vi "ExtendedKalmanFilter_New.vi"(5 "States":i32, 6 "UNSCENTED_KALMAN_FUNC_GROUP":T1, 7 "Inputs":i32, 8 "dt_Seconds":dbl=0.02, 9 "MeasurementStdDevs":T3, 10 "StateStdDevs":T3, 11 "Outputs":i32) -> (0 "Error":bool, 3 "UnscentedKalmanFiilter":T4)   [LabVIEW 2019, in "Trajectory_Library.lvlib"]
doc: "Creates a new LINEAR SYSTEM data cluster with the specified values. \n\n\nInputs: \n - XXX -- XXX.\n\nOutputs:\n - XXX -- XXX."
uses:
  Trajectory_Library.lvlib
  EXTENDED_KALMAN_FILTER.ctl
  <vilib>/Analysis/Matrix/Datatypes/RealMatrix.ctl
  EXTENDED_KALMAN_CORRECT_FUNC_GROUP.ctl
  BiFun_Matrix_FUNC_TYPE.ctl
  <vilib>/Analysis/7linalg.llb/Real Transpose Matrix.vi
  <vilib>/Analysis/baseanly.llb/A x B.vi
  <vilib>/Analysis/baseanly.llb/Real A x B.vi
  Discretization_DiscretizeA.vi
  <vilib>/Analysis/Matrix/Numeric/Add/Add.vi
  <vilib>/Analysis/Matrix/Numeric/Add/Add - RM,RM.vi
  <vilib>/Analysis/Matrix/Numeric/Multiply/Multiply.vi
  <vilib>/Analysis/Matrix/Numeric/Multiply/Multiply - RM,R.vi
  Matrix_Exp.vi
  <vilib>/Analysis/Matrix/NI_Matrix.lvlib
  <vilib>/Analysis/NI_AALPro.lvlib
panel:
  # "<States,1>"
  # "<Outputs,1>"
  # "State Estimate <Statess,1>"
  # "<States, States>"
  # "<States, States>"
  # "<Statess,  States>"
  # "<Outputs, Outputs>"
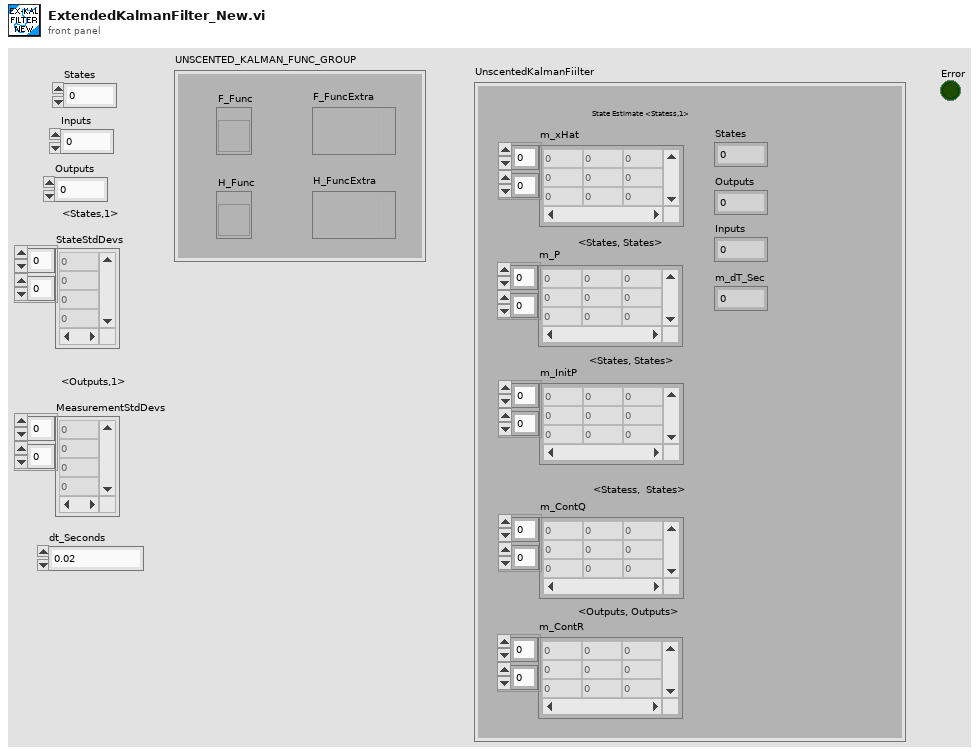
[diagram p1: front panel]
types:
  T1 = typedef "EXTENDED_KALMAN_CORRECT_FUNC_GROUP.ctl" = cluster{"H_Func":T2, "F_Func":T2, "H_FuncExtra":variant, "F_FuncExtra":variant}
  T2 = typedef "Trajectory_Library.lvlib/BiFun_Matrix_FUNC_TYPE.ctl" = refnum<vi>
  T3 = typedef "NI_Matrix.lvlib/RealMatrix.ctl" = dbl[][]
  T4 = typedef "Trajectory_Library.lvlib/EXTENDED_KALMAN_FILTER.ctl" = cluster{"m_P":T3, "m_xHat":T3, "States":i32, "Outputs":i32, "m_ContR":T3, "m_ContQ":T3, "m_dT_Sec":dbl, "Inputs":i32, "m_InitP":T3}
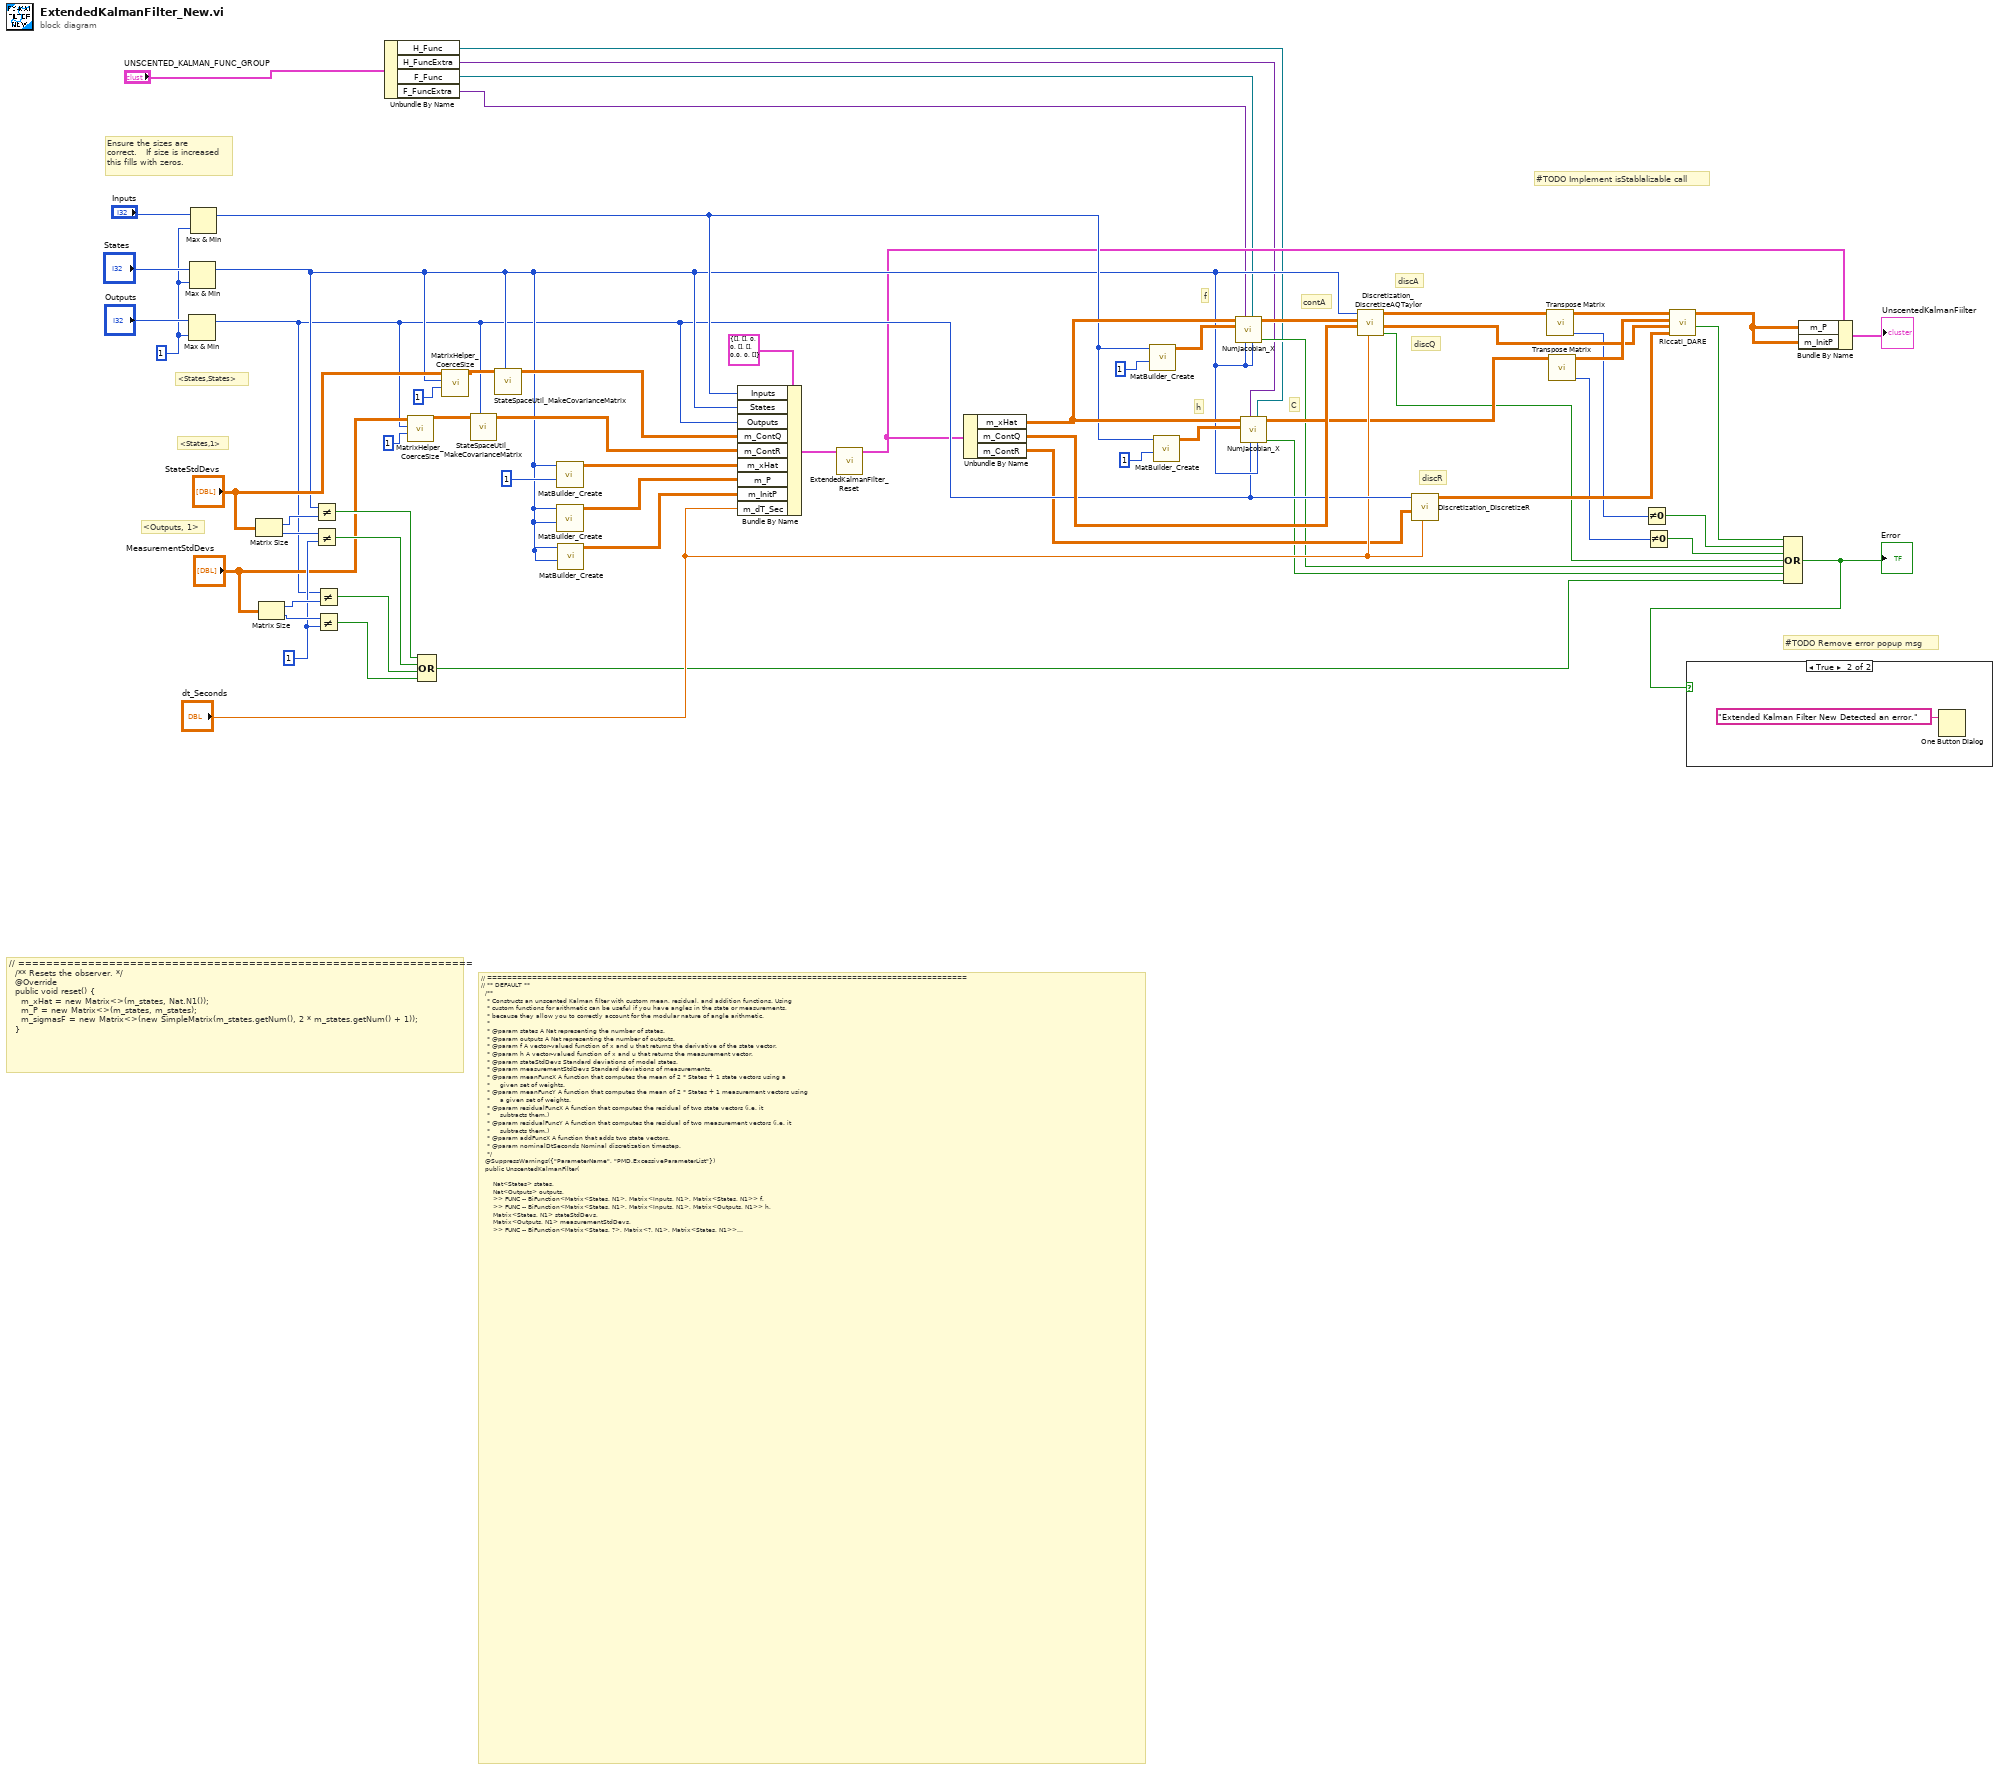
[diagram p0: block diagram]
diagram:
  w53 = 1 ("y")
  w47 = 1 ("y")
  # "#TODO Implement isStablalizable call"
  # "discR"
  # "discQ"
  # "discA"
  # "C"
  # "contA"
  # "h"
  # "f"
  # "// =================================================================\n  /** Resets the observer. */\n  @Override\n  public void reset() {\n    m_xHat = new Matrix<>(m_states, Nat.N1());\n    m_P = new Matrix<>(m_states, m_states);\n    m_sigmasF = new Matrix<>(new SimpleMatrix(m_states.getNum(), 2 * m_states.getNum() + 1));\n  }"
  # "// ================================================================================================\n// ** DEFAULT **\n  /**\n   * Constructs an unscented Kalman filter with custom mean, residual, and addition functions. Using\n   * custom functions for arithmetic can be useful if you have angles in the state or measurements,\n   * because they allow you to correctly account for the modular nature of angle arithmetic.\n   *\n   * @param states A Nat representing the number of states.\n   * @param outputs A Nat representing the number of outputs.\n   * @param f A vector-valued function of x and u that returns the derivative of the state vector.\n   * @param h A vector-valued function of x and u that returns the measurement vector.\n   * @param stateStdDevs Standard deviations of model states.\n   * @param measurementStdDevs Standard deviations of measurements.\n   * @param meanFuncX A function that computes the mean of 2 * States + 1 state vectors using a\n   *     given set of weights.\n   * @param meanFuncY A function that computes the mean of 2 * States + 1 measurement vectors using\n   *     a given set of weights.\n   * @param residualFuncX A function that computes the residual of two state vectors (i.e. it\n   *     subtracts them.)\n   * @param residualFuncY A function that computes the residual of two measurement vectors (i.e. it\n   *     subtracts them.)\n   * @param addFuncX A function that adds two state vectors.\n   * @param nominalDtSeconds Nominal discretization timestep.\n   */\n  @SuppressWarnings({\"ParameterName\", \"PMD.ExcessiveParameterList\"})\n  public UnscentedKalmanFilter(\n\n      Nat<States> states,\n      Nat<Outputs> outputs,\n      >> FUNC -- BiFunction<Matrix<States, N1>, Matrix<Inputs, N1>, Matrix<States, N1>> f,\n      >> FUNC -- BiFunction<Matrix<States, N1>, Matrix<Inputs, N1>, Matrix<Outputs, N1>> h,\n      Matrix<States, N1> stateStdDevs,\n      Matrix<Outputs, N1> measurementStdDevs,\n      >> FUNC -- BiFunction<Matrix<States, ?>, Matrix<?, N1>, Matrix<States, N1>> meanFuncX,\n      >> FUNC -- BiFunction<Matrix<Outputs, ?>, Matrix<?, N1>, Matrix<Outputs, N1>> meanFuncY,\n      >> FUNC -- BiFunction<Matrix<States, N1>, Matrix<States, N1>, Matrix<States, N1>> residualFuncX,\n      >> FUNC -- BiFunction<Matrix<Outputs, N1>, Matrix<Outputs, N1>, Matrix<Outputs, N1>> residualFuncY,\n      >> FUNC -- BiFunction<Matrix<States, N1>, Matrix<States, N1>, Matrix<States, N1>> addFuncX,\n      double nominalDtSeconds) {\n\n    this.m_states = states;\n    this.m_outputs = outputs;\n\n    m_f = f;\n    m_h = h;\n\n    m_meanFuncX = meanFuncX;\n    m_meanFuncY = meanFuncY;\n    m_residualFuncX = residualFuncX;\n    m_residualFuncY = residualFuncY;\n    m_addFuncX = addFuncX;\n\n    m_dtSeconds = nominalDtSeconds;\n\n    m_contQ = StateSpaceUtil.makeCovarianceMatrix(states, stateStdDevs);\n    m_contR = StateSpaceUtil.makeCovarianceMatrix(outputs, measurementStdDevs);\n\n    m_pts = new MerweScaledSigmaPoints<>(states);\n\n    reset();\n  }"
  # "#TODO Remove error popup msg"
  # "<Outputs, 1>"
  # "<States,1>"
  # "<States,States>"
  # "Ensure the sizes are\ncorrect.   If size is increased \nthis fills with zeros."
  n1 = Max & Min(x="Outputs", y=w47) -> (max(x,y)=w27:i32)  [unwired: 1 out]
  n2 = Max & Min(x="States", y=w47) -> (max(x,y)=w28:i32)  [unwired: 1 out]
  n3 = Max & Min(x="Inputs", y=w47) -> (max(x,y)=w32:i32)  [unwired: 1 out]
  n4 = Matrix Size(0:"StateStdDevs") -> (1:w61:i32, 2:w58:i32)
  n5 = Matrix Size(0:"MeasurementStdDevs") -> (1:w59:i32, 2:w60:i32)
  n6 = Not Equal?(x=w28, y=w61) -> (x != y?=w54:bool)
  n7 = Not Equal?(x=w58, y=w53) -> (x != y?=w55:bool)
  n8 = Not Equal?(x=w27, y=w59) -> (x != y?=w56:bool)
  n9 = Not Equal?(x=w60, y=w53) -> (x != y?=w57:bool)
  n10 = Unbundle By Name("UNSCENTED_KALMAN_FUNC_GROUP") -> ("H_Func"=w1:T2, "H_FuncExtra"=w2:variant, "F_Func"=w3:T2, "F_FuncExtra"=w4:variant)
  n11 = call "MatrixHelper_CoerceSize.vi"("Columns"=1, "Rows"=w27, "input matrix"="MeasurementStdDevs") -> ("output matrix"=w42:T3)  [unwired: 8 in]
  n12 = Compound Arithmetic op=OR(w54, w55, w56, w57) -> (w7:bool)
  n13 = call "MatrixHelper_CoerceSize.vi"("Columns"=1, "Rows"=w28, "input matrix"="StateStdDevs") -> ("output matrix"=w41:T3)  [unwired: 8 in]
  n14 = call "StateSpaceUtil_MakeCovarianceMatrix.vi"("States"=w27, "StdDevs"=w42) -> ("Covariance Matrix"=w45:T3)  [unwired: 9 in]
  n15 = call "StateSpaceUtil_MakeCovarianceMatrix.vi"("States"=w28, "StdDevs"=w41) -> ("Covariance Matrix"=w44:T3)  [unwired: 9 in]
  n16 = call "MatBuilder_Create.vi"("Columns"=1, "Rows"=w28) -> ("output matrix"=w50:T3)  [unwired: 9 in]
  n17 = call "MatBuilder_Create.vi"("Columns"=w28, "Rows"=w28) -> ("output matrix"=w49:T3)  [unwired: 9 in]
  n18 = call "MatBuilder_Create.vi"("Columns"=w28, "Rows"=w28) -> ("output matrix"=w43:T3)  [unwired: 9 in]
  n19 = Bundle By Name(cluster=T4 {"m_P"=[], "m_xHat"=[], "States"=0, "Outputs"=0, "m_ContR"=[], "m_ContQ"=[], "m_dT_Sec"=0.0, "Inputs"=0, "m_InitP"=[]} ("EXTENDED_KALMAN_FILTER"), "Inputs"=w32, "States"=w28, "Outputs"=w27, "m_ContQ"=w44, "m_ContR"=w45, "m_xHat"=w50, "m_P"=w49, "m_InitP"=w43, "m_dT_Sec"="dt_Seconds") -> (w46:T4)
  n20 = call "ExtendedKalmanFilter_Reset.vi"("in ExtendedKalmanFiilter"=w46) -> ("out ExtendedKalmanFiilter"=w18:T4)  [unwired: 10 in]
  n21 = Unbundle By Name(w18) -> ("m_xHat"=w34:T3, "m_ContQ"=w29:T3, "m_ContR"=w25:T3)
  n22 = call "MatBuilder_Create.vi"("Columns"=1, "Rows"=w32) -> ("output matrix"=w35:T3)  [unwired: 9 in]
  n23 = call "MatBuilder_Create.vi"("Columns"=1, "Rows"=w32) -> ("output matrix"=w31:T3)  [unwired: 9 in]
  n24 = call "NumJacobian_X.vi"("States"=w28, "F_FUNC"=w3, "Rows"=w28, "ExtraPassedData"=w4, "U"=w35, "X"=w34) -> ("Error"=w9:bool, "Result"=w30:T3)  [unwired: 4 in]
  n25 = call "NumJacobian_X.vi"("States"=w28, "F_FUNC"=w1, "Rows"=w27, "ExtraPassedData"=w2, "U"=w31, "X"=w34) -> ("Error"=w8:bool, "Result"=w23:T3)  [unwired: 4 in]
  n26 = call "Discretization_DiscretizeAQTaylor.vi"("dT_Seconds"="dt_Seconds", "ContQ"=w29, "ContA"=w30, "States"=w28) -> ("Error"=w10:bool, "DiscQ"=w20:T3, "DiscA"=w24:T3)  [unwired: 5 in]
  n27 = call "Discretization_DiscretizeR.vi"("dT_Seconds"="dt_Seconds", "ContR"=w25, "Outputs"=w27) -> ("DiscR"=w19:T3)  [unwired: 8 in]
  n28 = call-poly <vilib>:"Transpose Matrix.vi"("Input Matrix"=w24) -> ("error"=w14:i32, "Matrix Transpose"=w22:T3)  [unwired: 9 in]
  n29 = call-poly <vilib>:"Transpose Matrix.vi"("Input Matrix"=w23) -> ("error"=w13:i32, "Matrix Transpose"=w21:T3)  [unwired: 9 in]
  n30 = Not Equal To 0?(x=w14) -> (x != 0?=w12:bool)
  n31 = Not Equal To 0?(x=w13) -> (x != 0?=w11:bool)
  n32 = call "Riccati_DARE.vi"("R"=w19, "Q"=w20, "B"=w21, "A"=w22) -> ("Error"=w15:bool, "Answer"=w17:T3)  [unwired: 5 in, 1 out]
  n33 = Compound Arithmetic op=OR(w15, w12, w11, w10, w9, w8, w7) -> (w6:bool)
  "Error" <- w6
  n34 = case shown="True" w6 {
    frame False {
    }
    frame True {
      n35 = One Button Dialog(message="Extended Kalman Filter New Detected an error.") -> ()  [unwired: 1 in, 1 out]
    }
  }
  n36 = Bundle By Name(cluster=w18, "m_P"=w17, "m_InitP"=w17) -> (→"UnscentedKalmanFiilter":T4)
